vi "OnOffController.vi"(8 "histeresis":dbl, 9 "set_point":dbl, 10 "temp":dbl, 11 "u_k-1":bool) -> (3 "u_k":bool)   [LabVIEW 2020]
doc: "On/Off controller with histeresis."
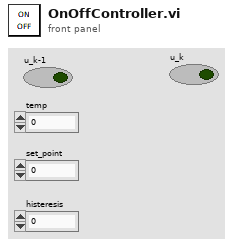
[diagram p1: front panel]
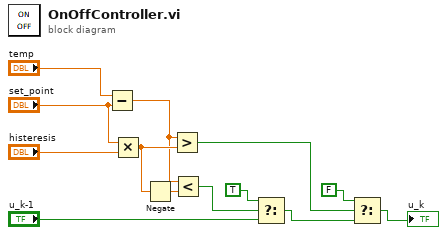
[diagram p0: block diagram]
diagram:
  n1 = Subtract(x="temp", y="set_point") -> (x-y=w7:dbl)
  n2 = Multiply(x="set_point", y="histeresis") -> (x*y=w9:dbl)
  n3 = Negate(x=w9) -> (-x=w8:dbl)
  n4 = Greater?(x=w7, y=w9) -> (0:w4:bool)
  n5 = Less?(x=w7, y=w8) -> (x < y?=w11:bool)
  n6 = Select(t=TRUE ("x > y?"), s=w11, f="u_k-1") -> (s? t:f=w12:bool)
  n7 = Select(t=FALSE ("x > y?"), s=w4, f=w12) -> (s? t:f=→"u_k":bool)
